vi "Offset Rectangle.vi"(10 "offset":T2, 11 "rect in":T1) -> (3 "rect out":T1)   [LabVIEW 2019]
doc: "Generate a new rectangle at the specified offset."
uses:
  <vilib>/Utility/miscctls.llb/LVPoint32TypeDef.ctl
  <vilib>/Utility/miscctls.llb/LVRectTypeDef.ctl
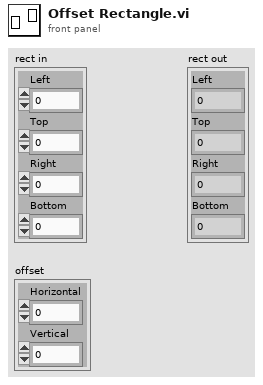
[diagram p1: front panel]
types:
  T1 = typedef "LVRectTypeDef.ctl" = cluster{"Left":i16, "Top":i16, "Right":i16, "Bottom":i16}
  T2 = typedef "LVPoint32TypeDef.ctl" = cluster{"Horizontal":i32, "Vertical":i32}
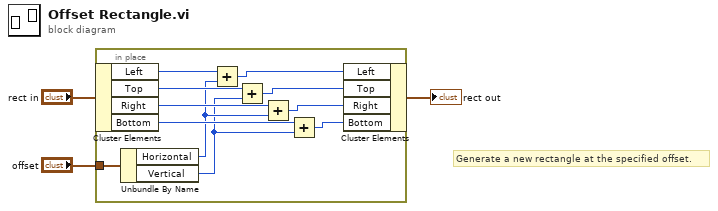
[diagram p0: block diagram]
diagram:
  # "Generate a new rectangle at the specified offset."
  n1 = in-place "In Place Element Structure" {
    in-place-border: "offset" -> [w10]
    n2 = in-place-cluster #1 ("Unbundle / Bundle Elements")("rect in") -> ("Left"=w14:i16, "Top"=w13:i16, "Right"=w12:i16, "Bottom"=w11:i16)
    n3 = Unbundle By Name(w10) -> ("Horizontal"=w9:i32, "Vertical"=w8:i32)
    n4 = Add(x=w14, y=w9) -> (x+y=w4:i32)
    n5 = Add(x=w13, y=w8) -> (x+y=w5:i32)
    n6 = Add(x=w12, y=w9) -> (x+y=w6:i32)
    n7 = Add(x=w11, y=w8) -> (x+y=w7:i32)
    n8 = in-place-cluster #1 ("Unbundle / Bundle Elements")("Left"=w4, "Top"=w5, "Right"=w6, "Bottom"=w7) -> (→"rect out":T1)
  }
